vi "AFP_increment.vi"(8 "AFP Min":i32, 9 "Sweep Direction":u16(ring), 10 "AFP Max":i32, 11 "AFP Target":i32) -> (3 "AFP Target Out":i32)   [LabVIEW 2018]
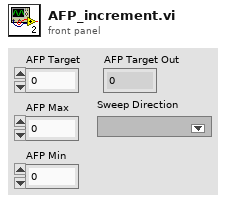
[diagram p1: front panel]
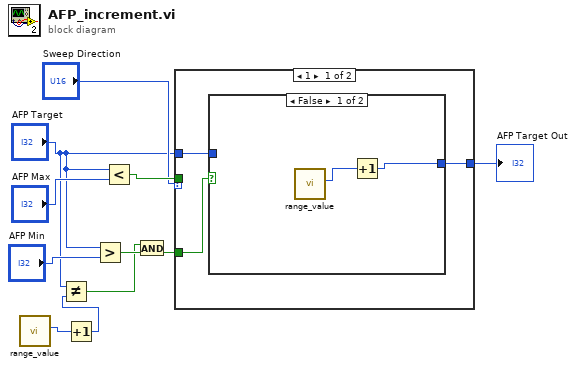
[diagram p0: block diagram]
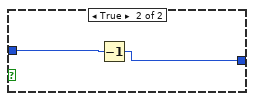
[diagram p2: hidden frame]
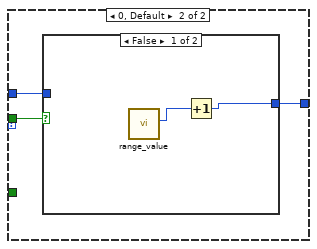
[diagram p3: hidden frame]
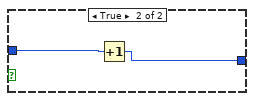
[diagram p4: hidden frame]
diagram:
  n1 = call "range_value.vi"() -> ("NumBins"=w3:i32)  [unwired: 10 in, 1 out]
  n2 = Increment(x=w3) -> (x+1=w2:i32)
  n3 = Not Equal?(x="AFP Target", y=w2) -> (x != y?=w4:bool)
  n4 = Greater?(x="AFP Target", y="AFP Min") -> (0:w6:bool)
  n5 = Less?(x="AFP Target", y="AFP Max") -> (x < y?=w10:bool)
  n6 = And(x=w4, y=w6) -> (x .and. y?=w5:bool)
  n7 = case shown="1" "Sweep Direction" {
    tunnel: w10 -> [_ w21]
    tunnel: "AFP Target" -> [w14 w20]
    tunnel: [w13 w19] -> w9
    tunnel: w5 -> [w12 _]
    frame 1 {
      n8 = case shown="False" w12 {
        tunnel: w14 -> [_ w18]
        tunnel: [w15 w17] -> w13
        frame False {
          n9 = call "range_value.vi"() -> ("NumBins"=w16:i32)  [unwired: 10 in, 1 out]
          n10 = Increment(x=w16) -> (x+1=w15:i32)
        }
        frame True {
          n11 = Decrement(x=w18) -> (x-1=w17:i32)
        }
      }
    }
    frame 0, Default {
      n12 = case shown="False" w21 {
        tunnel: w20 -> [_ w25]
        tunnel: [w22 w24] -> w19
        frame False {
          n13 = call "range_value.vi"() -> ("NumBins"=w23:i32)  [unwired: 10 in, 1 out]
          n14 = Increment(x=w23) -> (x+1=w22:i32)
        }
        frame True {
          n15 = Increment(x=w25) -> (x+1=w24:i32)
        }
      }
    }
  }
  "AFP Target Out" <- w9
